vi "Write Config Unitest.vi"(8 "error in (no error)":errorcluster, 11 "main ref":T1) -> (0 "error out":errorcluster)   [LabVIEW 2025]
uses:
  controls/LAB-IQ UI Data.ctl
  Config file  FGV Unitest enum.ctl
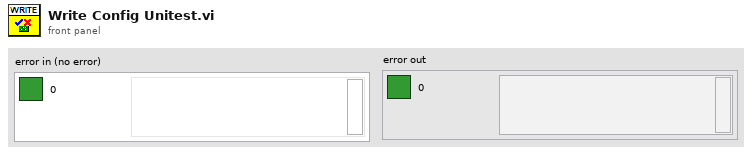
[diagram p1: front panel]
types:
  T1 = typedef "LAB-IQ UI Data.ctl" = cluster{"Main Home Screen":cluster{"GUI":refnum<vi>, "Platform Settings":refnum<vi>, "Configure":refnum<vi>, "Home":refnum<vi>, "EXIT":refnum<vi>, "service 2":refnum<vi>, "MainPage":refnum<vi>, "Analysis":refnum<vi>}, "Platform Settings":cluster{"mm/s  Surge":refnum<vi>, "Update Surge Speed":refnum<vi>, "Drive Error":refnum<vi>, "Disable Axis Jog Soft Limits":refnum<vi>, "mm/s  Sway":refnum<vi>, "Sway and Surge COM Status":refnum<vi>, "Heave COM Status":refnum<vi>, "Enable Platform":refnum<vi>, "Surge Forward Main":refnum<vi>, "Sway Right Main":refnum<vi>, "Sway Left Main":refnum<vi>, "Heave Down Main":refnum<vi>, "Heave Up main":refnum<vi>, "Update Sway Speed":refnum<vi>, "Update Heave Speed":refnum<vi>, "mm/s Heave":refnum<vi>, "mm/sec":refnum<vi>, "mm":refnum<vi>, "Surge Backward Main":refnum<vi>}, "Analysis Screen":cluster{"Analysis Home":refnum<vi>, "Surface Analysis":refnum<vi>, "Imaging":refnum<vi>, "Image Analysis":refnum<vi>, "Post Analysis":refnum<vi>}, "Config Screen":cluster{"Select Load Head":refnum<vi>, "Notes :":refnum<vi>, "FILE":refnum<vi>, "Sample ID :":refnum<vi>, "Operator ID :":refnum<vi>, "Operator Name :":refnum<vi>, "Auto":refnum<vi>}, "Motion Module":cluster{"zNL":refnum<vi>, "NL disp":refnum<vi>, "Rotary Tab":refnum<vi>, "Motion Direction:  3":refnum<vi>, "E.Velocity 2":refnum<vi>, "e.v/ssr 2":refnum<vi>, "Enter Fixed E.Velocity 2":refnum<vi>, "Enter Final SRR 2":refnum<vi>, "Enter initial SRR 2":refnum<vi>, "Enter Fixed SRR 2":refnum<vi>, "Enter the Final E.Velocity (m/s) 2":refnum<vi>, "Enter initial E.Velocity (m/s) 2":refnum<vi>, "Final Speed (RPM) 3":refnum<vi>, "Initial Speed (RPM) 2":refnum<vi>, "Enter the Final Velocity (m/s) 3":refnum<vi>, "Enter initial Velocity (m/s)  3":refnum<vi>, "Ramp Up 2":refnum<vi>, "TEST SELECTION":refnum<vi>, "SPEED SELECTION : ":refnum<vi>, "Angular Oscillation Set":refnum<vi>, "Traction":refnum<vi>, "Step Speed":refnum<vi>, "StepTable For Load-Speed":refnum<vi>, "StepTable For Speed":refnum<vi>, "Surge Forward MM":refnum<vi>, "Surge Backward MM":refnum<vi>, "M3 Image":refnum<vi>, "String 39":refnum<vi>, "Sway Left MM":refnum<vi>, "Sway Right MM":refnum<vi>, "Disable Axis Jog Soft Limits":refnum<vi>, "mm":refnum<vi>, "Heave Down MM":refnum<vi>, "Heave Up MM":refnum<vi>, "Wear Track Diameter (mm)":refnum<vi>, "Set WTD":refnum<vi>, "HomeScratch":refnum<vi>, "HomeRot":refnum<vi>, "PlaceModule":refnum<vi>, "Enter the Angle (Deg)":refnum<vi>, "Enter the Frequency (Hz)":refnum<vi>, "Motion Mode:":refnum<vi>, "LR Sway":refnum<vi>, "Rot Hor":refnum<vi>, "Scratch":refnum<vi>, "LR Cam":refnum<vi>, "MMBack":refnum<vi>, "MMNext":refnum<vi>, "Rot Ver":refnum<vi>, "Rotary Module Selection":refnum<vi>, "calculate rotary":refnum<vi>, "SPEED SELECTION : rotary":refnum<vi>, "Import 2":refnum<vi>, "Save 2":refnum<vi>, "File Path :  2":refnum<vi>, "String 45":refnum<vi>, "StepTable For Speed 3":refnum<vi>, "Enter the Speed(mm/sec)":refnum<vi>, "Enter the Speed(RPM)":refnum<vi>, "Enter Scratch Speed (mm/s):":refnum<vi>, "SwaySpeed Set":refnum<vi>, "Scartch Offset":refnum<vi>, "Motion type:":refnum<vi>, "HomeScratch 2":refnum<vi>, "Enter Scratch length (mm):":refnum<vi>, "Wear Track Diameter":refnum<vi>, "Rotary Speed Exced":refnum<vi>, "Scratch Mode":refnum<vi>, "No of Scratch":refnum<vi>}, "Environmental control":cluster{"Humidity  Status  3":refnum<vi>, "Low Temp  Status  2":refnum<vi>, "TK4 status 2":refnum<vi>, "Stage Temperature":refnum<vi>, "Sample Temperature":refnum<vi>, "Humidity (Amb)":refnum<vi>, "Clear List":refnum<vi>, "Add to list":refnum<vi>, "Wear":refnum<vi>, "Vibration":refnum<vi>, "Humidity (Chamber)":refnum<vi>, "Temperature (Chamber)":refnum<vi>, "ECR ":refnum<vi>, "Temperature (Amb)":refnum<vi>, "Microphone":refnum<vi>, "Acoustic Emission 3":refnum<vi>, "SNext":refnum<vi>, "APBack":refnum<vi>, "Enter the Temperature (°C):":refnum<vi>, "Enter the Stage \nTemperature (°C):":refnum<vi>, "Enter the Humidity (%Rh):":refnum<vi>, "Low Temp":refnum<vi>, "High Temp":refnum<vi>, "Humidity":refnum<vi>, "Sensors Picked":refnum<vi>}, "About Screen":cluster{"Password":refnum<vi>, "Home Service":refnum<vi>, "Advanced Setting":refnum<vi>, "About Tab":refnum<vi>, "ECR Port:":refnum<vi>, "Ramp Port:":refnum<vi>, "Installation/Replacement completed":refnum<vi>, "Loahead":refnum<vi>, "Heave and Surge COM Port:":refnum<vi>, "Sway COM Port:":refnum<vi>, "Temp Modbus:":refnum<vi>, "Humidity Port:":refnum<vi>, "Edit Gain Constants":refnum<vi>, "Save Gain Constants":refnum<vi>}, "Main Screen":cluster{"Main Screen Tab":refnum<vi>, "Angle and Frequency":refnum<vi>, "Stroke (mm)":refnum<vi>, "Angle (Deg)":refnum<vi>, "Main Speed Tab":refnum<vi>, "MTM MOTOR DISPLAY":refnum<vi>, "Disc Speed (m/sec)":refnum<vi>, "Ball Speed (m/sec)":refnum<vi>, "Disc Speed (RPM)":refnum<vi>, "Ball Speed (RPM)":refnum<vi>, "SPEED TAB":refnum<vi>, "Speed (m/sec)":refnum<vi>, "Set Speed (m/sec)":refnum<vi>, "Speed (RPM)":refnum<vi>, "Set Speed":refnum<vi>, "Time Tab":refnum<vi>, "Time ( HH:MM:SS ) 2":refnum<vi>, "Test Duration":refnum<vi>, "Test Duration 4":refnum<vi>, "TEST CYCLE":refnum<vi>, "TOTAL CYCLES":refnum<vi>, "Set Load (N)":refnum<vi>, "Temp Tabs":refnum<vi>, "Heater":refnum<vi>, "TK4 status":refnum<vi>, "ChamberTemp":refnum<vi>, "SetTmp":refnum<vi>, "Controller  Status":refnum<vi>, "ChamberTemp 2":refnum<vi>, "SetTmp 2":refnum<vi>, "Controller  Status 2":refnum<vi>, "ChamberTemp 3":refnum<vi>, "SetTmp 3":refnum<vi>, "Cooling":refnum<vi>, "Load Communication":refnum<vi>, "Ambient \nTemperature":refnum<vi>, "HumCOMStatus":refnum<vi>, "Ambient\n Humidity":refnum<vi>, "Freq (Hz)":refnum<vi>, "Load En":refnum<vi>, "NLt":refnum<vi>, "zNL 2":refnum<vi>, "Humidity On":refnum<vi>, "humidity disp":refnum<vi>, "Set Humidity":refnum<vi>, "NL disp 2":refnum<vi>, "Humidity On 2":refnum<vi>, "humidity disp 2":refnum<vi>, "Set Humidity 2":refnum<vi>, "NL disp 3":refnum<vi>, "AppLoadSeq scratch":refnum<vi>, "Stop Scratch":refnum<vi>, "ClrLog":refnum<vi>, "Trip Log":refnum<vi>, "STOP":refnum<vi>, "Start Test":refnum<vi>, "Test status":refnum<vi>, "AR Led":refnum<vi>, "Data":refnum<vi>, "Health":refnum<vi>, "Sway COM Status":refnum<vi>, "Heave COM Status":refnum<vi>, "Grp Tab":refnum<vi>, "Sub Graph":refnum<vi>, "SD (mm)":refnum<vi>, "Siliding distance Reset Graph":refnum<vi>, "SDGp":refnum<vi>, "Humidity Reset Graph":refnum<vi>, "HumrGp":refnum<vi>, "Acoustic Emission (mV)":refnum<vi>, "Aqucostic Reset Graph":refnum<vi>, "gACQUOS":refnum<vi>, "ECR RESET":refnum<vi>, "ECR":refnum<vi>, "Temperature Reset":refnum<vi>, "Acoustic Emission (mV) 2":refnum<vi>, "Aqucostic Reset Graph 2":refnum<vi>, "gACQUOS 2":refnum<vi>, "ECR RESET 2":refnum<vi>, "ECR 2":refnum<vi>, "Temperature Reset 2":refnum<vi>, "Temperature (deg c)":refnum<vi>, "Speed Reset Graph":refnum<vi>, "Speed Tab":refnum<vi>, "MTM DISC  SPEED":refnum<vi>, "MTM BALL SPEED":refnum<vi>, "speed mm/sec":refnum<vi>, "Hymidity":refnum<vi>, "Humidity Disable trip":refnum<vi>, "CoF Trip  2":refnum<vi>, "Depth Trip":refnum<vi>, "Weart Deapth":refnum<vi>, "Depth Reset Graph":refnum<vi>, "Weart":refnum<vi>, "Depthz":refnum<vi>, "Depth (µm)":refnum<vi>, "WearGp":refnum<vi>, "NL Trip 2":refnum<vi>, "Load pid":refnum<vi>, "Load Disable Trip":refnum<vi>, "Load Reset Graph":refnum<vi>, "NL Display 4":refnum<vi>, "Main Chart 3":refnum<vi>, "BACK":refnum<vi>, "Depth Trip 2":refnum<vi>, "COF TRIP ":refnum<vi>, "Friction Force (N)":refnum<vi>, "FF Reset Graph":refnum<vi>, "FF Disable Trip":refnum<vi>, "FF TRIP":refnum<vi>, "COF Disable Trip":refnum<vi>, "COF Reset Graph":refnum<vi>, "Start Test Temp":refnum<vi>, "zFF":refnum<vi>, "Friction Force (N) Graph":refnum<vi>, "Coefficient of Friction":refnum<vi>, "Scratch Start Test":refnum<vi>, "FF Tab":refnum<vi>, "Cyclic Friction Force (N)":refnum<vi>, "CZ FF":refnum<vi>, "Cyclic Friction Force (N) Graph":refnum<vi>, "Cyclic Coefficient of Friction":refnum<vi>, "Cyclic FF TRIP":refnum<vi>, "Cyclic FF Disable Trip":refnum<vi>, "cyclic COF Disable Trip":refnum<vi>, "cyclic COF TRIP":refnum<vi>, "cyclic COF Reset Graph":refnum<vi>, "Cyclic FF Reset Graph":refnum<vi>, "Test Trip":refnum<vi>, "Multi Scratch Pass":refnum<vi>, "Scratch Start Recording":refnum<vi>}, "Loading":cluster{"Indentation":refnum<vi>, "Reference Sample":refnum<vi>, "Load Cell Communication Slide":refnum<vi>, "com 3":refnum<vi>, "com":refnum<vi>, "DecaForce COM Status":refnum<vi>, "Update":refnum<vi>, "Clear 3":refnum<vi>, "seq":refnum<vi>, "Stribeck table":refnum<vi>, "Stribeck Table  For loading":refnum<vi>, "Loading Mode":refnum<vi>, "Enter the Final Load (N)":refnum<vi>, "Enter the CoF Trip":refnum<vi>, "Enter the Friction Force Trip":refnum<vi>, "Enter the Normal load Trip":refnum<vi>, "Enter the Load  (N)":refnum<vi>, "KiloForce":refnum<vi>, "DecaForce ":refnum<vi>, "MicroForce":refnum<vi>, "LHBack":refnum<vi>, "LHNext":refnum<vi>, "Enter the Loading Rate (N/min)":refnum<vi>, "Message":refnum<vi>, "Warning 2":refnum<vi>, "SSP 0.75":refnum<vi>, "SSP 0.5":refnum<vi>, "SSP 0.3":refnum<vi>, "Warning":refnum<vi>, "gui GIF":refnum<vi>, "Communication is established":refnum<vi>, "AppLoad 4":refnum<vi>, "Multipoint":refnum<vi>, "Load Selection":refnum<vi>}, "PID":cluster{"Ramp MulFac":refnum<vi>, "pulses LoadDiffRamp(2..10)":refnum<vi>, "PulseControlRamp(diff<=3N)":refnum<vi>, "SetLoadDeadband(%) Load(0-10N)":refnum<vi>, "PID gains out delay (microForce)":refnum<vi>, "Ramp":refnum<vi>, "Gain 2":refnum<vi>, "pulses LoadDiff(2..10)":refnum<vi>, "pulses LoadDiff(11..50)":refnum<vi>, "PulseControl(diff<=3N)":refnum<vi>, "SetLoadDeadband(%)  2":refnum<vi>, "Dummy Run":refnum<vi>, "Vertical load (N)":refnum<vi>, "AutoTune":refnum<vi>, "Offset 3 ":refnum<vi>, "apply load":refnum<vi>, "Offset  3":refnum<vi>, "apply load 2":refnum<vi>, "Enter ByPass Load":refnum<vi>, "reinit 3":refnum<vi>, "output range delay":refnum<vi>, "PID gains out delay":refnum<vi>, "Bypass Load":refnum<vi>, "pulsesSent":refnum<vi>, "pulses ":refnum<vi>, "actpid":refnum<vi>, "gFF Rot":refnum<vi>, "pulses LoadDiff(21..1000)":refnum<vi>, "Delay":refnum<vi>, "deadband":refnum<vi>}, "Config Parameters":cluster{"Tab Control 3":refnum<vi>, "Tab Control 19":refnum<vi>, "SAMPLES":refnum<vi>, "Re-initilaize":refnum<vi>, "Filter ON/OFF":refnum<vi>, "TracHomeSurgeOffsetCounts 10MM":refnum<vi>, "TracHomeSwayOffsetCounts 10MM":refnum<vi>, "Acoustic Emission:":refnum<vi>, "Apply Filter (FF)":refnum<vi>, "Filter% 2":refnum<vi>, "Apply Filter (Load)":refnum<vi>, "Filter% ":refnum<vi>, "Sway distance (mm)":refnum<vi>, "Surge distance (mm)":refnum<vi>, "DataSavingLoopDelay(ms)":refnum<vi>, "SAVE 2":refnum<vi>, "Enter Distance":refnum<vi>, "Sway Counts:":refnum<vi>, "Distance (mm): 3":refnum<vi>, "Surge Counts:":refnum<vi>, "Distance (mm): 2":refnum<vi>, "Distance (mm):":refnum<vi>, "Heave Counts:":refnum<vi>, "LRMHomeSurgeOffsetCounts":refnum<vi>, "LRMHomeSwayOffsetCounts":refnum<vi>, "TracHomeSurgeOffsetCounts 20MM":refnum<vi>, "TracHomeSwayOffsetCounts 20MM":refnum<vi>, "RotHomeSwayOffsetCounts":refnum<vi>, "RotHomeSurgeOffsetCounts":refnum<vi>, "Heave distance":refnum<vi>, "Zmm":refnum<vi>, "Heave Pulses/mm":refnum<vi>, "Surge Pulses/mm":refnum<vi>, "Sway Pulses/mm":refnum<vi>, "Heave Pitch":refnum<vi>, "Surge Pitch":refnum<vi>, "Sway Pitch":refnum<vi>, "Heave PPR":refnum<vi>, "Surge PPR":refnum<vi>, "Sway PPR":refnum<vi>, "Tab Control 5":refnum<vi>, "Tab Control 14":refnum<vi>, "Tab Control 26":refnum<vi>, "AE":refnum<vi>, "Heave Loop Delay":refnum<vi>, "Heave PID Speed":refnum<vi>, "Surge Jog Speed":refnum<vi>, "Heave Jog Speed":refnum<vi>, "Sway Loop Delay":refnum<vi>, "Sway PID Speed":refnum<vi>, "Sway Jog Speed":refnum<vi>, "DEPTH TRIP VALUE":refnum<vi>, "LOAD TRIP VALUE":refnum<vi>, "DEPTH TRIP   ENABLE":refnum<vi>, "LOAD TRIP  ENABLE":refnum<vi>, "CYCLIC FF TRIP VALUE":refnum<vi>, "FF TRIP VALUE":refnum<vi>, "CYCLIC CoF TRIP VALUE":refnum<vi>, "COF TRIP VALUE":refnum<vi>, "CYCLIC COF TRIP  ENABLE":refnum<vi>, "CYCLIC FF TRIP  ENABLE":refnum<vi>, "FF TRIP  ENABLE":refnum<vi>, "COF TRIP  ENABLE":refnum<vi>}, "Loading Com Port":cluster{"ClearAll":refnum<vi>, "Mz(Nm)":refnum<vi>, "My(Nm)":refnum<vi>, "Mx(Nm)":refnum<vi>, "Save Dwell":refnum<vi>, "Mx ":refnum<vi>, "My ":refnum<vi>, "Mz":refnum<vi>, "Fx(N)":refnum<vi>, "Fy(N)":refnum<vi>, "Fz(N)":refnum<vi>, "ZeroAll":refnum<vi>, "Acq Delay (ms)":refnum<vi>, "Burst Delay (ms)":refnum<vi>, "model":refnum<vi>, "SN":refnum<vi>, "FFx(N)":refnum<vi>, "Sensor IP":refnum<vi>, "Port":refnum<vi>, "FFy(N)":refnum<vi>, "Load(N)":refnum<vi>, "delete Handle":refnum<vi>, "Create Handle":refnum<vi>, "ft_data":refnum<vi>, "ft_range":refnum<vi>, "ft_data 2":refnum<vi>, "stop 6":refnum<vi>, "running_flag":refnum<vi>, "ft_udp_handle":refnum<vi>, "get-data-return":refnum<vi>, "get-range-return":refnum<vi>, "zero-return":refnum<vi>, "filter-return":refnum<vi>, "initial-return":refnum<vi>, "deleteHandle-result":refnum<vi>, "Load Cell Temp":refnum<vi>}, "Heave AND Surge":cluster{"SURGE POSE":refnum<vi>, "error out Read":refnum<vi>, "HEAVE POSE":refnum<vi>, "State":refnum<vi>, "Homed":refnum<vi>, "Sequence ID":refnum<vi>, "error out Write":refnum<vi>, "faultCode":refnum<vi>, "Ack ID":refnum<vi>, "SPEED":refnum<vi>, "Distance":refnum<vi>, "Mode Command":refnum<vi>, "Heave and Surge Read":refnum<vi>, "Read Heave Temp":refnum<vi>, "Spare 15":refnum<vi>, "Spare 14":refnum<vi>, "Spare 13":refnum<vi>, "Spare 12":refnum<vi>, "Spare 11":refnum<vi>, "Spare 10":refnum<vi>, "Spare 9":refnum<vi>, "Spare 8":refnum<vi>, "Spare 7":refnum<vi>, "Spare 6":refnum<vi>, "Spare 5":refnum<vi>, "Spare 4":refnum<vi>, "Spare 2":refnum<vi>, "Spare 1":refnum<vi>, "Node Id":refnum<vi>, "Spare 3":refnum<vi>, "SPARE 4":refnum<vi>, "SPARE 3":refnum<vi>, "SPARE 2":refnum<vi>, "SPARE 1":refnum<vi>, "fwMajor":refnum<vi>, "fwMinor":refnum<vi>, "Manual Write":refnum<vi>, "Heave and Surge Write":refnum<vi>}, "New PID LOGIC":cluster{"Fine Tune Zone":refnum<vi>, "PID SDelay":refnum<vi>, "Max_pos_limit":refnum<vi>, "Min_pos_limit":refnum<vi>, "i_limit":refnum<vi>, "pct_scale":refnum<vi>, "Deadband":refnum<vi>, "Kd":refnum<vi>, "Ki":refnum<vi>, "Kp":refnum<vi>, "Current Position":refnum<vi>, "Set Load":refnum<vi>, "Current Load":refnum<vi>, "Pulse delta":refnum<vi>, "Init Step":refnum<vi>, "Max Step Linit":refnum<vi>}, "SWAY ":cluster{"fwMajor":refnum<vi>, "Homed":refnum<vi>, "Rotary POSE":refnum<vi>, "State":refnum<vi>, "SWAY POSE":refnum<vi>, "Ack ID":refnum<vi>, "faultCode":refnum<vi>, "Node Id":refnum<vi>, "fwMinor":refnum<vi>, "Spare 6":refnum<vi>, "Spare 5":refnum<vi>, "Spare 4":refnum<vi>, "Spare 3":refnum<vi>, "Spare 2":refnum<vi>, "Spare 1":refnum<vi>, "Spare 7":refnum<vi>, "SPARE  5":refnum<vi>, "error out Write  SWAY ":refnum<vi>, "error out Read SWAY ":refnum<vi>, "Manual Write SWAY ":refnum<vi>, "SWAY WRITE":refnum<vi>, "SPARE  4":refnum<vi>, "SPARE  3":refnum<vi>, "SPARE 2":refnum<vi>, "SPARE 1":refnum<vi>, "Spare 15":refnum<vi>, "Spare 14":refnum<vi>, "Spare 13":refnum<vi>, "Spare 12":refnum<vi>, "Spare 11":refnum<vi>, "Spare 9":refnum<vi>, "Spare 8":refnum<vi>, "SPEED":refnum<vi>, "Distance":refnum<vi>, "Mode Command":refnum<vi>, "Sequence ID":refnum<vi>, "SWAY READ":refnum<vi>, "Spare 10":refnum<vi>, "Read SWAY Temp":refnum<vi>}, "Analysis Screen":cluster{"Analysis Home":refnum<vi>, "Refresh 2":refnum<vi>, "MEAN 4":refnum<vi>, "SD 4":refnum<vi>, "VARIANCE 4":refnum<vi>, "MEAN  3":refnum<vi>, "SD  3":refnum<vi>, "VARIANCE  3":refnum<vi>, "MEAN 2":refnum<vi>, "SD  2":refnum<vi>, "VARIANCE 2":refnum<vi>, "MEAN":refnum<vi>, "SD":refnum<vi>, "VARIANCE":refnum<vi>, "File 4 Discription":refnum<vi>, "OPEN 4":refnum<vi>, "File Name 4":refnum<vi>, "OPEN 3":refnum<vi>, "File 3 Discription":refnum<vi>, "File Name 3":refnum<vi>, "Y-AXIS":refnum<vi>, "X-AXIS":refnum<vi>, "XY Graph":refnum<vi>, "File Name 2":refnum<vi>, "File Name 1":refnum<vi>, "OPEN 2":refnum<vi>, "OPEN 1":refnum<vi>, "File 1 Discription ":refnum<vi>, "File 2 Discription":refnum<vi>, "Export":refnum<vi>, "File Format":refnum<vi>}}
  T2 = typedef "Config file  FGV Unitest enum.ctl" = enum16{"OPEN", "READ", "WRITE", "CLOSE"}
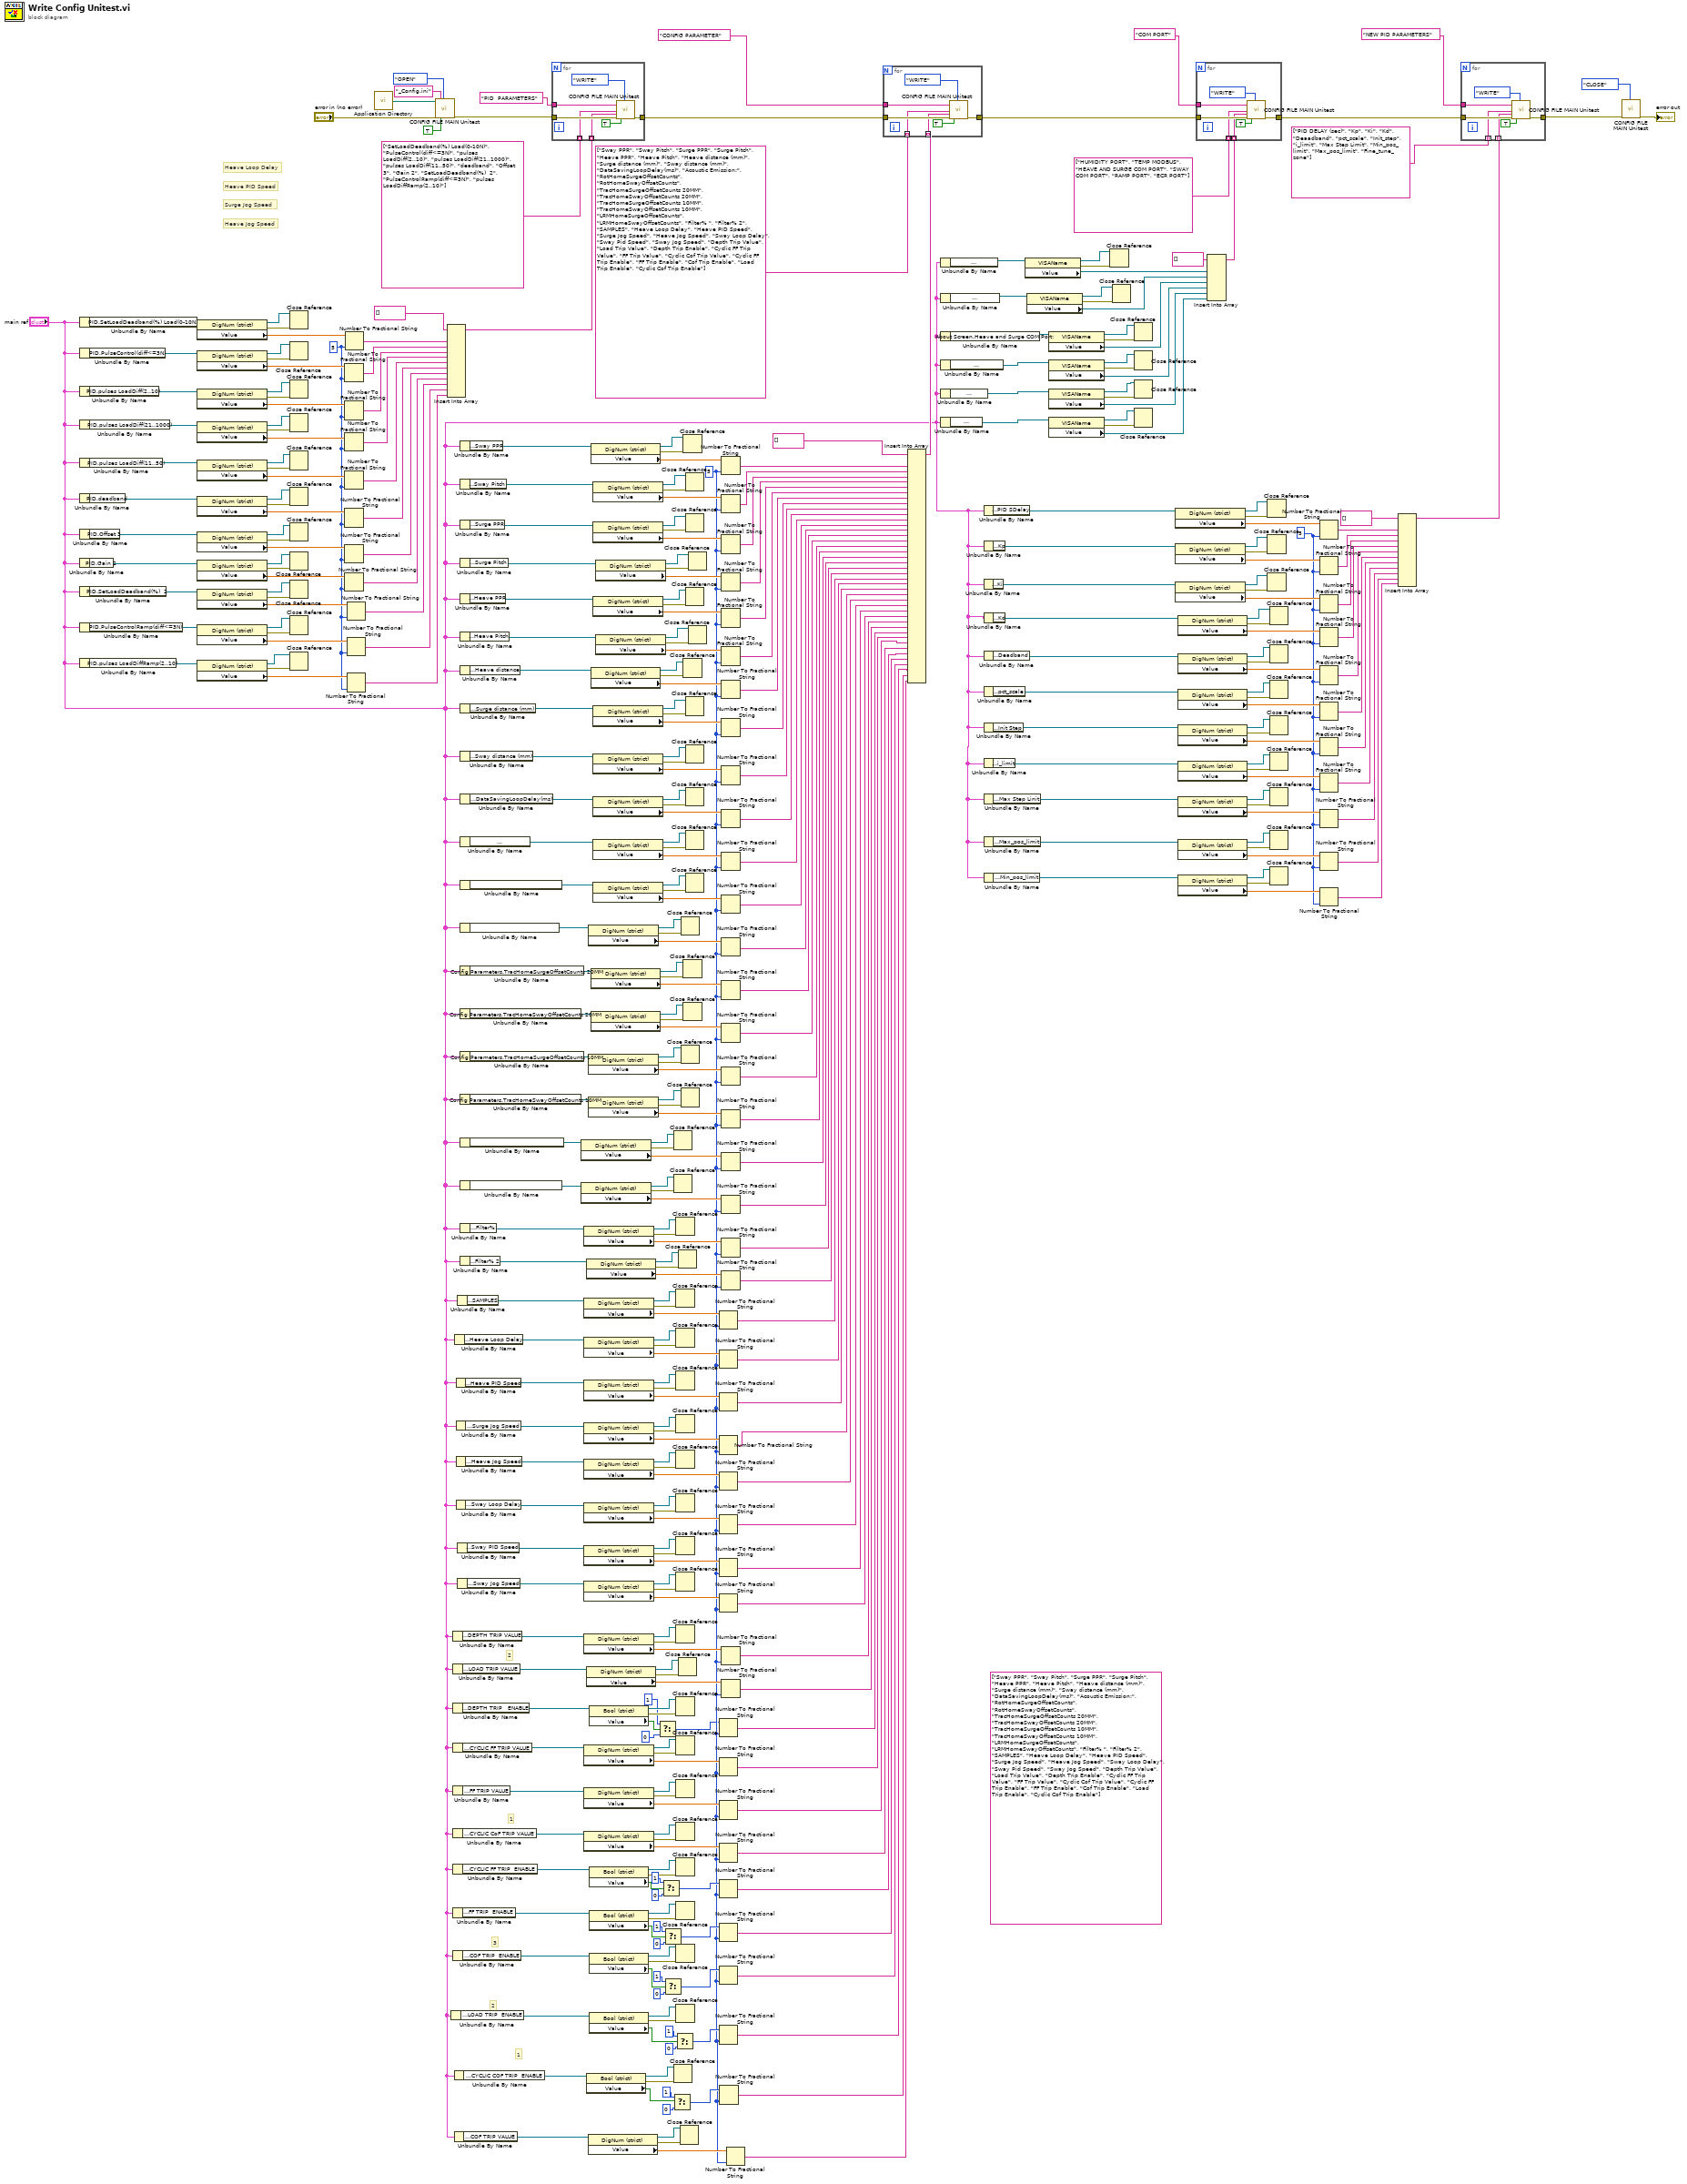
[diagram p0: block diagram]
diagram:
  (unwired) string[] ["Sway PPR", "Sway Pitch", "Surge PPR", "Surge Pitch", "Heave PPR", "Heave Pitch", "Heave distance (mm)", "Surge distance (mm)", "Sway distance (mm)", "DataSavingLoopDelay(ms)", "Acoustic Emission:", "RotHomeSurgeOffsetCounts", "RotHomeSwayOffsetCounts", "TracHomeSurgeOffsetCounts 20MM", "TracHomeSwayOffsetCounts 20MM", "TracHomeSurgeOffsetCounts 10MM", "TracHomeSwayOffsetCounts 10MM", "LRMHomeSurgeOffsetCounts", "LRMHomeSwayOffsetCounts", "Filter% ", "Filter% 2", "SAMPLES", "Heave Loop Delay", "Heave PID Speed", "Surge Jog Speed", "Heave Jog Speed", "Sway Loop Delay", "Sway Pid Speed", "Sway Jog Speed", "Depth Trip Value", "Load Trip Value", "Depth Trip Enable", "Cyclic FF Trip Value", "FF Trip Value", "Cyclic Cof Trip Value", "Cyclic FF Trip Enable", "FF Trip Enable", "Cof Trip Enable", "Load Trip Enable", "Cyclic Cof Trip Enable"]
  w110 = i16 5 ("precision (6)")
  w4 = i16 5 ("precision (6)")
  w329 = i16 5 ("precision (6)")
  # "3"
  # "2"
  # "2"
  # "1"
  # "1"
  # "Heave Jog Speed"
  # "Surge Jog Speed"
  # "Heave PID Speed"
  # "Heave Loop Delay"
  n1 = Unbundle By Name("main ref") -> ("PID.SetLoadDeadband(%) Load(0-10N)"=w373:refnum<vi>)
  n2 = Unbundle By Name("main ref") -> ("PID.PulseControl(diff<=3N)"=w368:refnum<vi>)
  n3 = Unbundle By Name("main ref") -> ("PID.pulses LoadDiff(2..10)"=w367:refnum<vi>)
  n4 = Unbundle By Name("main ref") -> ("PID.pulses LoadDiff(21..1000)"=w362:refnum<vi>)
  n5 = Unbundle By Name("main ref") -> ("PID.pulses LoadDiff(11..50)"=w361:refnum<vi>)
  n6 = Unbundle By Name("main ref") -> ("PID.deadband"=w356:refnum<vi>)
  n7 = Unbundle By Name("main ref") -> ("PID.Offset 3"=w355:refnum<vi>)
  n8 = Unbundle By Name("main ref") -> ("PID.Gain 2"=w350:refnum<vi>)
  n9 = Unbundle By Name("main ref") -> ("PID.SetLoadDeadband(%)  2"=w349:refnum<vi>)
  n10 = Unbundle By Name("main ref") -> ("PID.PulseControlRamp(diff<=3N)"=w345:refnum<vi>)
  n11 = Unbundle By Name("main ref") -> ("PID.pulses LoadDiffRamp(2..10)"=w343:refnum<vi>)
  n12 = property class="DigNum (strict)"(reference=w373) -> (reference out=w371:refnum<vi>, error out=w372:errorcluster, "Value"=w339:dbl)  [unwired: 1 in]
  n13 = property class="DigNum (strict)"(reference=w368) -> (reference out=w370:refnum<vi>, error out=w369:errorcluster, "Value"=w340:dbl)  [unwired: 1 in]
  n14 = property class="DigNum (strict)"(reference=w367) -> (reference out=w365:refnum<vi>, error out=w366:errorcluster, "Value"=w338:dbl)  [unwired: 1 in]
  n15 = property class="DigNum (strict)"(reference=w362) -> (reference out=w364:refnum<vi>, error out=w363:errorcluster, "Value"=w337:dbl)  [unwired: 1 in]
  n16 = property class="DigNum (strict)"(reference=w361) -> (reference out=w359:refnum<vi>, error out=w360:errorcluster, "Value"=w336:dbl)  [unwired: 1 in]
  n17 = property class="DigNum (strict)"(reference=w356) -> (reference out=w358:refnum<vi>, error out=w357:errorcluster, "Value"=w335:dbl)  [unwired: 1 in]
  n18 = property class="DigNum (strict)"(reference=w355) -> (reference out=w353:refnum<vi>, error out=w354:errorcluster, "Value"=w334:dbl)  [unwired: 1 in]
  n19 = property class="DigNum (strict)"(reference=w350) -> (reference out=w352:refnum<vi>, error out=w351:errorcluster, "Value"=w333:dbl)  [unwired: 1 in]
  n20 = property class="DigNum (strict)"(reference=w349) -> (reference out=w347:refnum<vi>, error out=w348:errorcluster, "Value"=w332:dbl)  [unwired: 1 in]
  n21 = property class="DigNum (strict)"(reference=w345) -> (reference out=w344:refnum<vi>, error out=w346:errorcluster, "Value"=w331:dbl)  [unwired: 1 in]
  n22 = property class="DigNum (strict)"(reference=w343) -> (reference out=w341:refnum<vi>, error out=w342:errorcluster, "Value"=w330:dbl)  [unwired: 1 in]
  n23 = Close Reference(reference=w371, error in (no error)=w372) -> ()  [unwired: 1 out]
  n24 = Close Reference(reference=w370, error in (no error)=w369) -> ()  [unwired: 1 out]
  n25 = Close Reference(reference=w365, error in (no error)=w366) -> ()  [unwired: 1 out]
  n26 = Close Reference(reference=w364, error in (no error)=w363) -> ()  [unwired: 1 out]
  n27 = Close Reference(reference=w359, error in (no error)=w360) -> ()  [unwired: 1 out]
  n28 = Close Reference(reference=w358, error in (no error)=w357) -> ()  [unwired: 1 out]
  n29 = Close Reference(reference=w353, error in (no error)=w354) -> ()  [unwired: 1 out]
  n30 = Close Reference(reference=w352, error in (no error)=w351) -> ()  [unwired: 1 out]
  n31 = Close Reference(reference=w347, error in (no error)=w348) -> ()  [unwired: 1 out]
  n32 = Close Reference(reference=w344, error in (no error)=w346) -> ()  [unwired: 1 out]
  n33 = Close Reference(reference=w341, error in (no error)=w342) -> ()  [unwired: 1 out]
  n34 = Number To Fractional String(number=w340, precision (6)=w329) -> (F-format string=w326:string)  [unwired: 2 in]
  n35 = Number To Fractional String(number=w338, precision (6)=w329) -> (F-format string=w325:string)  [unwired: 2 in]
  n36 = Number To Fractional String(number=w337, precision (6)=w329) -> (F-format string=w324:string)  [unwired: 2 in]
  n37 = Number To Fractional String(number=w336, precision (6)=w329) -> (F-format string=w323:string)  [unwired: 2 in]
  n38 = Number To Fractional String(number=w335, precision (6)=w329) -> (F-format string=w322:string)  [unwired: 2 in]
  n39 = Number To Fractional String(number=w334, precision (6)=w329) -> (F-format string=w321:string)  [unwired: 2 in]
  n40 = Number To Fractional String(number=w333, precision (6)=w329) -> (F-format string=w320:string)  [unwired: 2 in]
  n41 = Number To Fractional String(number=w339, precision (6)=w329) -> (F-format string=w327:string)  [unwired: 2 in]
  n42 = Number To Fractional String(number=w332, precision (6)=w329) -> (F-format string=w319:string)  [unwired: 2 in]
  n43 = Number To Fractional String(number=w331, precision (6)=w329) -> (F-format string=w318:string)  [unwired: 2 in]
  n44 = Number To Fractional String(number=w330, precision (6)=w329) -> (F-format string=w317:string)  [unwired: 2 in]
  n45 = call <vilib>:"Application Directory.vi"() -> ("Application Directory"=w385:path)
  n46 = call "CONFIG FILE MAIN Unitest.vi"("File Path"=w385, "error in"="error in (no error)", "file name"="_Config.ini", "PARAMETER/CONFIG"=TRUE, "Config Enum"=Config_file__FGV_Unitest_enum."OPEN") -> ("error out"=w384:errorcluster)  [unwired: 13 in, 1 out]
  n47 = Insert Into Array(array=string[] [], new element #1=w327, new element #2=w326, new element #3=w325, new element #4=w324, new element #5=w323, new element #6=w322, new element #7=w321, new element #8=w320, new element #9=w319, new element #10=w318, new element #11=w317) -> (w316:string[])  [unwired: 1 in]
  n48 = Unbundle By Name("main ref") -> ("Config Parameters.LOAD TRIP  ENABLE"=w46:refnum<vi>)
  n49 = Unbundle By Name("main ref") -> ("Config Parameters.DEPTH TRIP VALUE"=w50:refnum<vi>)
  n50 = Unbundle By Name("main ref") -> ("Config Parameters.LOAD TRIP VALUE"=w56:refnum<vi>)
  n51 = Unbundle By Name("main ref") -> ("Config Parameters.DEPTH TRIP   ENABLE"=w57:refnum<vi>)
  n52 = Unbundle By Name("main ref") -> ("Config Parameters.CYCLIC FF TRIP VALUE"=w64:refnum<vi>)
  n53 = Unbundle By Name("main ref") -> ("Config Parameters.FF TRIP VALUE"=w65:refnum<vi>)
  n54 = Unbundle By Name("main ref") -> ("Config Parameters.CYCLIC CoF TRIP VALUE"=w72:refnum<vi>)
  n55 = Unbundle By Name("main ref") -> ("Config Parameters.CYCLIC FF TRIP  ENABLE"=w73:refnum<vi>)
  n56 = Unbundle By Name("main ref") -> ("Config Parameters.FF TRIP  ENABLE"=w81:refnum<vi>)
  n57 = Unbundle By Name("main ref") -> ("Config Parameters.COF TRIP  ENABLE"=w76:refnum<vi>)
  n58 = Unbundle By Name("main ref") -> ("Config Parameters.CYCLIC COF TRIP  ENABLE"=w31:refnum<vi>)
  n59 = Unbundle By Name("main ref") -> ("Config Parameters.COF TRIP VALUE"=w9:refnum<vi>)
  n60 = Unbundle By Name("main ref") -> ("Config Parameters.Heave Loop Delay"=w175:refnum<vi>)
  n61 = Unbundle By Name("main ref") -> ("Config Parameters.Heave PID Speed"=w174:refnum<vi>)
  n62 = Unbundle By Name("main ref") -> ("Config Parameters.Surge Jog Speed"=w167:refnum<vi>)
  n63 = Unbundle By Name("main ref") -> ("Config Parameters.Heave Jog Speed"=w166:refnum<vi>)
  n64 = Unbundle By Name("main ref") -> ("Config Parameters.Sway Loop Delay"=w85:refnum<vi>)
  n65 = Unbundle By Name("main ref") -> ("Config Parameters.SAMPLES"=w233:refnum<vi>)
  n66 = Unbundle By Name("main ref") -> ("Config Parameters.Sway PID Speed"=w92:refnum<vi>)
  n67 = Unbundle By Name("main ref") -> ("Config Parameters.Sway Jog Speed"=w93:refnum<vi>)
  n68 = Unbundle By Name("main ref") -> ("Config Parameters.Sway PPR"=w315:refnum<vi>)
  n69 = Unbundle By Name("main ref") -> ("Config Parameters.Sway Pitch"=w308:refnum<vi>)
  n70 = Unbundle By Name("main ref") -> ("Config Parameters.Surge PPR"=w300:refnum<vi>)
  n71 = Unbundle By Name("main ref") -> ("Config Parameters.Surge Pitch"=w307:refnum<vi>)
  n72 = Unbundle By Name("main ref") -> ("Config Parameters.Heave PPR"=w299:refnum<vi>)
  n73 = Unbundle By Name("main ref") -> ("Config Parameters.Heave Pitch"=w293:refnum<vi>)
  n74 = Unbundle By Name("main ref") -> ("Config Parameters.Heave distance"=w285:refnum<vi>)
  n75 = Unbundle By Name("main ref") -> ("Config Parameters.Surge distance (mm)"=w291:refnum<vi>)
  n76 = Unbundle By Name("main ref") -> ("Config Parameters.Sway distance (mm)"=w282:refnum<vi>)
  n77 = Unbundle By Name("main ref") -> ("Config Parameters.DataSavingLoopDelay(ms)"=w279:refnum<vi>)
  n78 = Unbundle By Name("main ref") -> ("Config Parameters.Acoustic Emission:"=w274:refnum<vi>)
  n79 = Unbundle By Name("main ref") -> ("Config Parameters.RotHomeSurgeOffsetCounts"=w271:refnum<vi>)
  n80 = Unbundle By Name("main ref") -> ("Config Parameters.RotHomeSwayOffsetCounts"=w266:refnum<vi>)
  n81 = Unbundle By Name("main ref") -> ("Config Parameters.TracHomeSurgeOffsetCounts 20MM"=w263:refnum<vi>)
  n82 = Unbundle By Name("main ref") -> ("Config Parameters.TracHomeSwayOffsetCounts 20MM"=w258:refnum<vi>)
  n83 = Unbundle By Name("main ref") -> ("Config Parameters.TracHomeSurgeOffsetCounts 10MM"=w252:refnum<vi>)
  n84 = Unbundle By Name("main ref") -> ("Config Parameters.TracHomeSwayOffsetCounts 10MM"=w257:refnum<vi>)
  n85 = Unbundle By Name("main ref") -> ("Config Parameters.LRMHomeSurgeOffsetCounts"=w246:refnum<vi>)
  n86 = Unbundle By Name("main ref") -> ("Config Parameters.LRMHomeSwayOffsetCounts"=w241:refnum<vi>)
  n87 = Unbundle By Name("main ref") -> ("Config Parameters.Filter%"=w240:refnum<vi>)
  n88 = Unbundle By Name("main ref") -> ("Config Parameters.Filter% 2"=w234:refnum<vi>)
  n89 = for {
    tunnel: w384 -> [w396]
    tunnel: "PID  PARAMETERS" ("WRITE /READ SECTION") -> [w395]
    tunnel: string[] ["SetLoadDeadband(%) Load(0-10N)", "PulseControl(diff<=3N)", "pulses LoadDiff(2..10)", "pulses LoadDiff(21..1000)", "pulses LoadDiff(11..50)", "deadband", "Offset  3", "Gain 2", "SetLoadDeadband(%)  2", "PulseControlRamp(diff<=3N)", "pulses LoadDiffRamp(2..10)"] -> [w392] mode=indexing
    tunnel: [w394] -> w381
    tunnel: w316 -> [w391] mode=indexing
    n90 = call "CONFIG FILE MAIN Unitest.vi"("WRITE /READ SECTION"=w395, "WRITE KEY"=w392, "WRITE VALUE"=w391, "error in"=w396, "PARAMETER/CONFIG"=TRUE, "Config Enum"=Config_file__FGV_Unitest_enum."WRITE") -> ("error out"=w394:errorcluster)  [unwired: 12 in, 1 out]
  }
  n91 = property class="DigNum (strict)"(reference=w246) -> (reference out=w247:refnum<vi>, error out=w245:errorcluster, "Value"=w244:dbl)  [unwired: 1 in]
  n92 = property class="DigNum (strict)"(reference=w241) -> (reference out=w248:refnum<vi>, error out=w242:errorcluster, "Value"=w243:dbl)  [unwired: 1 in]
  n93 = property class="DigNum (strict)"(reference=w240) -> (reference out=w237:refnum<vi>, error out=w239:errorcluster, "Value"=w238:dbl)  [unwired: 1 in]
  n94 = property class="DigNum (strict)"(reference=w233) -> (reference out=w230:refnum<vi>, error out=w232:errorcluster, "Value"=w231:dbl)  [unwired: 1 in]
  n95 = property class="DigNum (strict)"(reference=w175) -> (reference out=w178:refnum<vi>, error out=w176:errorcluster, "Value"=w177:dbl)  [unwired: 1 in]
  n96 = property class="DigNum (strict)"(reference=w174) -> (reference out=w171:refnum<vi>, error out=w173:errorcluster, "Value"=w172:dbl)  [unwired: 1 in]
  n97 = property class="DigNum (strict)"(reference=w167) -> (reference out=w170:refnum<vi>, error out=w168:errorcluster, "Value"=w169:dbl)  [unwired: 1 in]
  n98 = property class="DigNum (strict)"(reference=w166) -> (reference out=w163:refnum<vi>, error out=w165:errorcluster, "Value"=w164:dbl)  [unwired: 1 in]
  n99 = property class="DigNum (strict)"(reference=w85) -> (reference out=w88:refnum<vi>, error out=w86:errorcluster, "Value"=w87:dbl)  [unwired: 1 in]
  n100 = property class="DigNum (strict)"(reference=w92) -> (reference out=w89:refnum<vi>, error out=w91:errorcluster, "Value"=w90:dbl)  [unwired: 1 in]
  n101 = property class="DigNum (strict)"(reference=w93) -> (reference out=w96:refnum<vi>, error out=w94:errorcluster, "Value"=w95:dbl)  [unwired: 1 in]
  n102 = property class="DigNum (strict)"(reference=w50) -> (reference out=w53:refnum<vi>, error out=w51:errorcluster, "Value"=w52:dbl)  [unwired: 1 in]
  n103 = property class="DigNum (strict)"(reference=w64) -> (reference out=w61:refnum<vi>, error out=w63:errorcluster, "Value"=w62:dbl)  [unwired: 1 in]
  n104 = property class="DigNum (strict)"(reference=w65) -> (reference out=w68:refnum<vi>, error out=w66:errorcluster, "Value"=w67:dbl)  [unwired: 1 in]
  n105 = property class="DigNum (strict)"(reference=w72) -> (reference out=w69:refnum<vi>, error out=w71:errorcluster, "Value"=w70:dbl)  [unwired: 1 in]
  n106 = property class="DigNum (strict)"(reference=w234) -> (reference out=w229:refnum<vi>, error out=w235:errorcluster, "Value"=w236:dbl)  [unwired: 1 in]
  n107 = property class="DigNum (strict)"(reference=w56) -> (reference out=w60:refnum<vi>, error out=w55:errorcluster, "Value"=w54:dbl)  [unwired: 1 in]
  n108 = property class="Bool (strict)"(reference=w31) -> (reference out=w33:refnum<vi>, error out=w32:errorcluster, "Value"=w22:bool)  [unwired: 1 in]
  n109 = property class="DigNum (strict)"(reference=w9) -> (reference out=w7:refnum<vi>, error out=w8:errorcluster, "Value"=w5:dbl)  [unwired: 1 in]
  n110 = property class="DigNum (strict)"(reference=w266) -> (reference out=w265:refnum<vi>, error out=w267:errorcluster, "Value"=w268:dbl)  [unwired: 1 in]
  n111 = property class="DigNum (strict)"(reference=w252) -> (reference out=w250:refnum<vi>, error out=w253:errorcluster, "Value"=w254:dbl)  [unwired: 1 in]
  n112 = property class="DigNum (strict)"(reference=w257) -> (reference out=w249:refnum<vi>, error out=w256:errorcluster, "Value"=w255:dbl)  [unwired: 1 in]
  n113 = property class="Bool (strict)"(reference=w57) -> (reference out=w59:refnum<vi>, error out=w58:errorcluster, "Value"=w49:bool)  [unwired: 1 in]
  n114 = property class="Bool (strict)"(reference=w73) -> (reference out=w75:refnum<vi>, error out=w74:errorcluster, "Value"=w27:bool)  [unwired: 1 in]
  n115 = property class="Bool (strict)"(reference=w81) -> (reference out=w79:refnum<vi>, error out=w80:errorcluster, "Value"=w28:bool)  [unwired: 1 in]
  n116 = property class="Bool (strict)"(reference=w76) -> (reference out=w78:refnum<vi>, error out=w77:errorcluster, "Value"=w29:bool)  [unwired: 1 in]
  n117 = property class="Bool (strict)"(reference=w46) -> (reference out=w44:refnum<vi>, error out=w45:errorcluster, "Value"=w30:bool)  [unwired: 1 in]
  n118 = property class="DigNum (strict)"(reference=w315) -> (reference out=w313:refnum<vi>, error out=w314:errorcluster, "Value"=w312:dbl)  [unwired: 1 in]
  n119 = property class="DigNum (strict)"(reference=w285) -> (reference out=w204:refnum<vi>, error out=w286:errorcluster, "Value"=w287:dbl)  [unwired: 1 in]
  n120 = property class="DigNum (strict)"(reference=w263) -> (reference out=w264:refnum<vi>, error out=w262:errorcluster, "Value"=w261:dbl)  [unwired: 1 in]
  n121 = property class="DigNum (strict)"(reference=w258) -> (reference out=w251:refnum<vi>, error out=w259:errorcluster, "Value"=w260:dbl)  [unwired: 1 in]
  n122 = property class="DigNum (strict)"(reference=w308) -> (reference out=w310:refnum<vi>, error out=w309:errorcluster, "Value"=w311:dbl)  [unwired: 1 in]
  n123 = property class="DigNum (strict)"(reference=w300) -> (reference out=w302:refnum<vi>, error out=w301:errorcluster, "Value"=w303:dbl)  [unwired: 1 in]
  n124 = property class="DigNum (strict)"(reference=w299) -> (reference out=w292:refnum<vi>, error out=w298:errorcluster, "Value"=w297:dbl)  [unwired: 1 in]
  n125 = property class="DigNum (strict)"(reference=w291) -> (reference out=w289:refnum<vi>, error out=w290:errorcluster, "Value"=w288:dbl)  [unwired: 1 in]
  n126 = property class="DigNum (strict)"(reference=w282) -> (reference out=w281:refnum<vi>, error out=w283:errorcluster, "Value"=w284:dbl)  [unwired: 1 in]
  n127 = property class="DigNum (strict)"(reference=w279) -> (reference out=w280:refnum<vi>, error out=w278:errorcluster, "Value"=w277:dbl)  [unwired: 1 in]
  n128 = property class="DigNum (strict)"(reference=w274) -> (reference out=w273:refnum<vi>, error out=w275:errorcluster, "Value"=w276:dbl)  [unwired: 1 in]
  n129 = property class="DigNum (strict)"(reference=w271) -> (reference out=w272:refnum<vi>, error out=w270:errorcluster, "Value"=w269:dbl)  [unwired: 1 in]
  n130 = property class="DigNum (strict)"(reference=w307) -> (reference out=w305:refnum<vi>, error out=w306:errorcluster, "Value"=w304:dbl)  [unwired: 1 in]
  n131 = property class="DigNum (strict)"(reference=w293) -> (reference out=w295:refnum<vi>, error out=w294:errorcluster, "Value"=w296:dbl)  [unwired: 1 in]
  n132 = Select(t=1, s=w49, f=0) -> (s? t:f=w1:i32)
  n133 = Select(t=1, s=w27, f=0) -> (s? t:f=w26:i32)
  n134 = Select(t=1, s=w28, f=0) -> (s? t:f=w25:i32)
  n135 = Select(t=1, s=w29, f=0) -> (s? t:f=w24:i32)
  n136 = Select(t=1, s=w22, f=0) -> (s? t:f=w21:i32)
  n137 = Close Reference(reference=w247, error in (no error)=w245) -> ()  [unwired: 1 out]
  n138 = Close Reference(reference=w248, error in (no error)=w242) -> ()  [unwired: 1 out]
  n139 = Close Reference(reference=w33, error in (no error)=w32) -> ()  [unwired: 1 out]
  n140 = Select(t=1, s=w30, f=0) -> (s? t:f=w23:i32)
  n141 = Close Reference(reference=w237, error in (no error)=w239) -> ()  [unwired: 1 out]
  n142 = Close Reference(reference=w230, error in (no error)=w232) -> ()  [unwired: 1 out]
  n143 = Close Reference(reference=w178, error in (no error)=w176) -> ()  [unwired: 1 out]
  n144 = Close Reference(reference=w171, error in (no error)=w173) -> ()  [unwired: 1 out]
  n145 = Close Reference(reference=w170, error in (no error)=w168) -> ()  [unwired: 1 out]
  n146 = Close Reference(reference=w163, error in (no error)=w165) -> ()  [unwired: 1 out]
  n147 = Close Reference(reference=w88, error in (no error)=w86) -> ()  [unwired: 1 out]
  n148 = Close Reference(reference=w89, error in (no error)=w91) -> ()  [unwired: 1 out]
  n149 = Close Reference(reference=w96, error in (no error)=w94) -> ()  [unwired: 1 out]
  n150 = Close Reference(reference=w53, error in (no error)=w51) -> ()  [unwired: 1 out]
  n151 = Close Reference(reference=w59, error in (no error)=w58) -> ()  [unwired: 1 out]
  n152 = Close Reference(reference=w61, error in (no error)=w63) -> ()  [unwired: 1 out]
  n153 = Close Reference(reference=w68, error in (no error)=w66) -> ()  [unwired: 1 out]
  n154 = Close Reference(reference=w69, error in (no error)=w71) -> ()  [unwired: 1 out]
  n155 = Close Reference(reference=w75, error in (no error)=w74) -> ()  [unwired: 1 out]
  n156 = Close Reference(reference=w79, error in (no error)=w80) -> ()  [unwired: 1 out]
  n157 = Close Reference(reference=w78, error in (no error)=w77) -> ()  [unwired: 1 out]
  n158 = Close Reference(reference=w44, error in (no error)=w45) -> ()  [unwired: 1 out]
  n159 = Close Reference(reference=w229, error in (no error)=w235) -> ()  [unwired: 1 out]
  n160 = Close Reference(reference=w60, error in (no error)=w55) -> ()  [unwired: 1 out]
  n161 = Close Reference(reference=w7, error in (no error)=w8) -> ()  [unwired: 1 out]
  n162 = Close Reference(reference=w265, error in (no error)=w267) -> ()  [unwired: 1 out]
  n163 = Close Reference(reference=w250, error in (no error)=w253) -> ()  [unwired: 1 out]
  n164 = Close Reference(reference=w249, error in (no error)=w256) -> ()  [unwired: 1 out]
  n165 = Close Reference(reference=w313, error in (no error)=w314) -> ()  [unwired: 1 out]
  n166 = Close Reference(reference=w204, error in (no error)=w286) -> ()  [unwired: 1 out]
  n167 = Close Reference(reference=w264, error in (no error)=w262) -> ()  [unwired: 1 out]
  n168 = Close Reference(reference=w251, error in (no error)=w259) -> ()  [unwired: 1 out]
  n169 = Close Reference(reference=w310, error in (no error)=w309) -> ()  [unwired: 1 out]
  n170 = Close Reference(reference=w302, error in (no error)=w301) -> ()  [unwired: 1 out]
  n171 = Close Reference(reference=w292, error in (no error)=w298) -> ()  [unwired: 1 out]
  n172 = Close Reference(reference=w289, error in (no error)=w290) -> ()  [unwired: 1 out]
  n173 = Close Reference(reference=w281, error in (no error)=w283) -> ()  [unwired: 1 out]
  n174 = Close Reference(reference=w280, error in (no error)=w278) -> ()  [unwired: 1 out]
  n175 = Close Reference(reference=w273, error in (no error)=w275) -> ()  [unwired: 1 out]
  n176 = Close Reference(reference=w272, error in (no error)=w270) -> ()  [unwired: 1 out]
  n177 = Close Reference(reference=w305, error in (no error)=w306) -> ()  [unwired: 1 out]
  n178 = Close Reference(reference=w295, error in (no error)=w294) -> ()  [unwired: 1 out]
  n179 = Number To Fractional String(number=w231, precision (6)=w4) -> (F-format string=w206:string)  [unwired: 2 in]
  n180 = Number To Fractional String(number=w177, precision (6)=w4) -> (F-format string=w162:string)  [unwired: 2 in]
  n181 = Number To Fractional String(number=w172, precision (6)=w4) -> (F-format string=w161:string)  [unwired: 2 in]
  n182 = Number To Fractional String(number=w169, precision (6)=w4) -> (F-format string=w160:string)  [unwired: 2 in]
  n183 = Number To Fractional String(number=w164, precision (6)=w4) -> (F-format string=w159:string)  [unwired: 2 in]
  n184 = Number To Fractional String(number=w87, precision (6)=w4) -> (F-format string=w84:string)  [unwired: 2 in]
  n185 = Number To Fractional String(number=w90, precision (6)=w4) -> (F-format string=w83:string)  [unwired: 2 in]
  n186 = Number To Fractional String(number=w95, precision (6)=w4) -> (F-format string=w82:string)  [unwired: 2 in]
  n187 = Number To Fractional String(number=w1, precision (6)=w4) -> (F-format string=w18:string)  [unwired: 2 in]
  n188 = Number To Fractional String(number=w62, precision (6)=w4) -> (F-format string=w17:string)  [unwired: 2 in]
  n189 = Number To Fractional String(number=w67, precision (6)=w4) -> (F-format string=w16:string)  [unwired: 2 in]
  n190 = Number To Fractional String(number=w70, precision (6)=w4) -> (F-format string=w15:string)  [unwired: 2 in]
  n191 = Number To Fractional String(number=w26, precision (6)=w4) -> (F-format string=w14:string)  [unwired: 2 in]
  n192 = Number To Fractional String(number=w25, precision (6)=w4) -> (F-format string=w13:string)  [unwired: 2 in]
  n193 = Number To Fractional String(number=w24, precision (6)=w4) -> (F-format string=w12:string)  [unwired: 2 in]
  n194 = Number To Fractional String(number=w23, precision (6)=w4) -> (F-format string=w11:string)  [unwired: 2 in]
  n195 = Number To Fractional String(number=w21, precision (6)=w4) -> (F-format string=w10:string)  [unwired: 2 in]
  n196 = Number To Fractional String(number=w312, precision (6)=w4) -> (F-format string=w227:string)  [unwired: 2 in]
  n197 = Number To Fractional String(number=w311, precision (6)=w4) -> (F-format string=w226:string)  [unwired: 2 in]
  n198 = Number To Fractional String(number=w303, precision (6)=w4) -> (F-format string=w225:string)  [unwired: 2 in]
  n199 = Number To Fractional String(number=w304, precision (6)=w4) -> (F-format string=w224:string)  [unwired: 2 in]
  n200 = Number To Fractional String(number=w297, precision (6)=w4) -> (F-format string=w223:string)  [unwired: 2 in]
  n201 = Number To Fractional String(number=w296, precision (6)=w4) -> (F-format string=w222:string)  [unwired: 2 in]
  n202 = Number To Fractional String(number=w287, precision (6)=w4) -> (F-format string=w221:string)  [unwired: 2 in]
  n203 = Number To Fractional String(number=w288, precision (6)=w4) -> (F-format string=w220:string)  [unwired: 2 in]
  n204 = Number To Fractional String(number=w284, precision (6)=w4) -> (F-format string=w219:string)  [unwired: 2 in]
  n205 = Number To Fractional String(number=w277, precision (6)=w4) -> (F-format string=w218:string)  [unwired: 2 in]
  n206 = Number To Fractional String(number=w276, precision (6)=w4) -> (F-format string=w217:string)  [unwired: 2 in]
  n207 = Number To Fractional String(number=w269, precision (6)=w4) -> (F-format string=w216:string)  [unwired: 2 in]
  n208 = Number To Fractional String(number=w268, precision (6)=w4) -> (F-format string=w215:string)  [unwired: 2 in]
  n209 = Number To Fractional String(number=w261, precision (6)=w4) -> (F-format string=w214:string)  [unwired: 2 in]
  n210 = Number To Fractional String(number=w260, precision (6)=w4) -> (F-format string=w213:string)  [unwired: 2 in]
  n211 = Number To Fractional String(number=w254, precision (6)=w4) -> (F-format string=w212:string)  [unwired: 2 in]
  n212 = Number To Fractional String(number=w255, precision (6)=w4) -> (F-format string=w211:string)  [unwired: 2 in]
  n213 = Number To Fractional String(number=w244, precision (6)=w4) -> (F-format string=w210:string)  [unwired: 2 in]
  n214 = Number To Fractional String(number=w243, precision (6)=w4) -> (F-format string=w209:string)  [unwired: 2 in]
  n215 = Number To Fractional String(number=w238, precision (6)=w4) -> (F-format string=w208:string)  [unwired: 2 in]
  n216 = Number To Fractional String(number=w236, precision (6)=w4) -> (F-format string=w207:string)  [unwired: 2 in]
  n217 = Number To Fractional String(number=w52, precision (6)=w4) -> (F-format string=w20:string)  [unwired: 2 in]
  n218 = Number To Fractional String(number=w54, precision (6)=w4) -> (F-format string=w19:string)  [unwired: 2 in]
  n219 = Number To Fractional String(number=w5, precision (6)=w4) -> (F-format string=w3:string)  [unwired: 2 in]
  n220 = Insert Into Array(array=string[] [], new element #1=w227, new element #2=w226, new element #3=w225, new element #4=w224, new element #5=w223, new element #6=w222, new element #7=w221, new element #8=w220, new element #9=w219, new element #10=w218, new element #11=w217, new element #12=w216, new element #13=w215, new element #14=w214, new element #15=w213, new element #16=w212, new element #17=w211, new element #18=w210, new element #19=w209, new element #20=w208, new element #21=w207, new element #22=w206, new element #23=w162, new element #24=w161, new element #25=w160, new element #26=w159, new element #27=w84, new element #28=w83, new element #29=w82, new element #30=w20, new element #31=w19, new element #32=w18, new element #33=w17, new element #34=w16, new element #35=w15, new element #36=w14, new element #37=w13, new element #38=w12, new element #39=w11, new element #40=w10, new element #41=w3) -> (w205:string[])  [unwired: 1 in]
  n221 = for {
    tunnel: w381 -> [w403]
    tunnel: "CONFIG PARAMETER" ("WRITE /READ SECTION") -> [w402]
    tunnel: [w401] -> w379
    tunnel: string[] ["Sway PPR", "Sway Pitch", "Surge PPR", "Surge Pitch", "Heave PPR", "Heave Pitch", "Heave distance (mm)", "Surge distance (mm)", "Sway distance (mm)", "DataSavingLoopDelay(ms)", "Acoustic Emission:", "RotHomeSurgeOffsetCounts", "RotHomeSwayOffsetCounts", "TracHomeSurgeOffsetCounts 20MM", "TracHomeSwayOffsetCounts 20MM", "TracHomeSurgeOffsetCounts 10MM", "TracHomeSwayOffsetCounts 10MM", "LRMHomeSurgeOffsetCounts", "LRMHomeSwayOffsetCounts", "Filter% ", "Filter% 2", "SAMPLES", "Heave Loop Delay", "Heave PID Speed", "Surge Jog Speed", "Heave Jog Speed", "Sway Loop Delay", "Sway Pid Speed", "Sway Jog Speed", "Depth Trip Value", "Load Trip Value", "Depth Trip Enable", "Cyclic FF Trip Value", "FF Trip Value", "Cyclic Cof Trip Value", "Cyclic FF Trip Enable", "FF Trip Enable", "Cof Trip Enable", "Load Trip Enable", "Cyclic Cof Trip Enable"] -> [w399] mode=indexing
    tunnel: w205 -> [w397] mode=indexing
    n222 = call "CONFIG FILE MAIN Unitest.vi"("WRITE /READ SECTION"=w402, "WRITE KEY"=w399, "WRITE VALUE"=w397, "error in"=w403, "PARAMETER/CONFIG"=TRUE, "Config Enum"=Config_file__FGV_Unitest_enum."WRITE") -> ("error out"=w401:errorcluster)  [unwired: 12 in, 1 out]
  }
  n223 = Unbundle By Name("main ref") -> ("About Screen.Humidity Port:"=w202:refnum<vi>)
  n224 = Unbundle By Name("main ref") -> ("About Screen.Temp Modbus:"=w197:refnum<vi>)
  n225 = Unbundle By Name("main ref") -> ("About Screen.Heave and Surge COM Port:"=w194:refnum<vi>)
  n226 = Unbundle By Name("main ref") -> ("About Screen.Sway COM Port:"=w190:refnum<vi>)
  n227 = Unbundle By Name("main ref") -> ("About Screen.Ramp Port:"=w189:refnum<vi>)
  n228 = Unbundle By Name("main ref") -> ("About Screen.ECR Port:"=w186:refnum<vi>)
  n229 = Unbundle By Name("main ref") -> ("New PID LOGIC.PID SDelay"=w152:refnum<vi>)
  n230 = Unbundle By Name("main ref") -> ("New PID LOGIC.Kp"=w151:refnum<vi>)
  n231 = Unbundle By Name("main ref") -> ("New PID LOGIC.Ki"=w146:refnum<vi>)
  n232 = Unbundle By Name("main ref") -> ("New PID LOGIC.Kd"=w145:refnum<vi>)
  n233 = Unbundle By Name("main ref") -> ("New PID LOGIC.Deadband"=w141:refnum<vi>)
  n234 = Unbundle By Name("main ref") -> ("New PID LOGIC.pct_scale"=w140:refnum<vi>)
  n235 = Unbundle By Name("main ref") -> ("New PID LOGIC.Init Step"=w137:refnum<vi>)
  n236 = Unbundle By Name("main ref") -> ("New PID LOGIC.i_limit"=w136:refnum<vi>)
  n237 = Unbundle By Name("main ref") -> ("New PID LOGIC.Max Step Linit"=w133:refnum<vi>)
  n238 = Unbundle By Name("main ref") -> ("New PID LOGIC.Max_pos_limit"=w131:refnum<vi>)
  n239 = Unbundle By Name("main ref") -> ("New PID LOGIC.Min_pos_limit"=w130:refnum<vi>)
  n240 = property class="VISAName"(reference=w202) -> (reference out=w200:refnum<vi>, error out=w201:errorcluster, "Value"=w196:refnum<visa-resource-name>)  [unwired: 1 in]
  n241 = property class="VISAName"(reference=w197) -> (reference out=w199:refnum<vi>, error out=w198:errorcluster, "Value"=w195:refnum<visa-resource-name>)  [unwired: 1 in]
  n242 = property class="VISAName"(reference=w194) -> (reference out=w192:refnum<vi>, error out=w193:errorcluster, "Value"=w185:refnum<visa-resource-name>)  [unwired: 1 in]
  n243 = property class="VISAName"(reference=w190) -> (reference out=w184:refnum<vi>, error out=w191:errorcluster, "Value"=w183:refnum<visa-resource-name>)  [unwired: 1 in]
  n244 = property class="VISAName"(reference=w189) -> (reference out=w180:refnum<vi>, error out=w188:errorcluster, "Value"=w182:refnum<visa-resource-name>)  [unwired: 1 in]
  n245 = property class="VISAName"(reference=w186) -> (reference out=w179:refnum<vi>, error out=w187:errorcluster, "Value"=w181:refnum<visa-resource-name>)  [unwired: 1 in]
  n246 = Close Reference(reference=w200, error in (no error)=w201) -> ()  [unwired: 1 out]
  n247 = Close Reference(reference=w199, error in (no error)=w198) -> ()  [unwired: 1 out]
  n248 = Close Reference(reference=w192, error in (no error)=w193) -> ()  [unwired: 1 out]
  n249 = Close Reference(reference=w184, error in (no error)=w191) -> ()  [unwired: 1 out]
  n250 = Close Reference(reference=w180, error in (no error)=w188) -> ()  [unwired: 1 out]
  n251 = Close Reference(reference=w179, error in (no error)=w187) -> ()  [unwired: 1 out]
  n252 = property class="DigNum (strict)"(reference=w152) -> (reference out=w154:refnum<vi>, error out=w153:errorcluster, "Value"=w121:dbl)  [unwired: 1 in]
  n253 = property class="DigNum (strict)"(reference=w151) -> (reference out=w149:refnum<vi>, error out=w150:errorcluster, "Value"=w120:dbl)  [unwired: 1 in]
  n254 = property class="DigNum (strict)"(reference=w146) -> (reference out=w148:refnum<vi>, error out=w147:errorcluster, "Value"=w119:dbl)  [unwired: 1 in]
  n255 = property class="DigNum (strict)"(reference=w145) -> (reference out=w143:refnum<vi>, error out=w144:errorcluster, "Value"=w118:dbl)  [unwired: 1 in]
  n256 = property class="DigNum (strict)"(reference=w141) -> (reference out=w127:refnum<vi>, error out=w142:errorcluster, "Value"=w117:dbl)  [unwired: 1 in]
  n257 = property class="DigNum (strict)"(reference=w140) -> (reference out=w128:refnum<vi>, error out=w139:errorcluster, "Value"=w116:dbl)  [unwired: 1 in]
  n258 = property class="DigNum (strict)"(reference=w137) -> (reference out=w126:refnum<vi>, error out=w138:errorcluster, "Value"=w115:dbl)  [unwired: 1 in]
  n259 = property class="DigNum (strict)"(reference=w136) -> (reference out=w125:refnum<vi>, error out=w135:errorcluster, "Value"=w114:dbl)  [unwired: 1 in]
  n260 = property class="DigNum (strict)"(reference=w133) -> (reference out=w124:refnum<vi>, error out=w134:errorcluster, "Value"=w113:dbl)  [unwired: 1 in]
  n261 = property class="DigNum (strict)"(reference=w131) -> (reference out=w123:refnum<vi>, error out=w132:errorcluster, "Value"=w112:dbl)  [unwired: 1 in]
  n262 = property class="DigNum (strict)"(reference=w130) -> (reference out=w122:refnum<vi>, error out=w129:errorcluster, "Value"=w111:dbl)  [unwired: 1 in]
  n263 = Insert Into Array(array=string[] [], new element #1=w196, new element #2=w195, new element #3=w185, new element #4=w183, new element #5=w182, new element #6=w181) -> (w375:string[])  [unwired: 1 in]
  n264 = for {
    tunnel: w379 -> [w410]
    tunnel: "COM PORT" ("WRITE /READ SECTION") -> [w409]
    tunnel: [w408] -> w156
    tunnel: string[] ["HUMIDITY PORT", "TEMP MODBUS", "HEAVE AND SURGE COM PORT", "SWAY COM PORT", "RAMP PORT", "ECR PORT"] -> [w406] mode=indexing
    tunnel: w375 -> [w405] mode=indexing
    n265 = call "CONFIG FILE MAIN Unitest.vi"("WRITE /READ SECTION"=w409, "WRITE KEY"=w406, "WRITE VALUE"=w405, "error in"=w410, "PARAMETER/CONFIG"=TRUE, "Config Enum"=Config_file__FGV_Unitest_enum."WRITE") -> ("error out"=w408:errorcluster)  [unwired: 12 in, 1 out]
  }
  n266 = Close Reference(reference=w154, error in (no error)=w153) -> ()  [unwired: 1 out]
  n267 = Close Reference(reference=w149, error in (no error)=w150) -> ()  [unwired: 1 out]
  n268 = Close Reference(reference=w148, error in (no error)=w147) -> ()  [unwired: 1 out]
  n269 = Close Reference(reference=w143, error in (no error)=w144) -> ()  [unwired: 1 out]
  n270 = Close Reference(reference=w127, error in (no error)=w142) -> ()  [unwired: 1 out]
  n271 = Close Reference(reference=w128, error in (no error)=w139) -> ()  [unwired: 1 out]
  n272 = Close Reference(reference=w126, error in (no error)=w138) -> ()  [unwired: 1 out]
  n273 = Close Reference(reference=w125, error in (no error)=w135) -> ()  [unwired: 1 out]
  n274 = Close Reference(reference=w124, error in (no error)=w134) -> ()  [unwired: 1 out]
  n275 = Close Reference(reference=w123, error in (no error)=w132) -> ()  [unwired: 1 out]
  n276 = Close Reference(reference=w122, error in (no error)=w129) -> ()  [unwired: 1 out]
  n277 = Number To Fractional String(number=w121, precision (6)=w110) -> (F-format string=w108:string)  [unwired: 2 in]
  n278 = Number To Fractional String(number=w120, precision (6)=w110) -> (F-format string=w107:string)  [unwired: 2 in]
  n279 = Number To Fractional String(number=w119, precision (6)=w110) -> (F-format string=w106:string)  [unwired: 2 in]
  n280 = Number To Fractional String(number=w118, precision (6)=w110) -> (F-format string=w105:string)  [unwired: 2 in]
  n281 = Number To Fractional String(number=w117, precision (6)=w110) -> (F-format string=w104:string)  [unwired: 2 in]
  n282 = Number To Fractional String(number=w116, precision (6)=w110) -> (F-format string=w103:string)  [unwired: 2 in]
  n283 = Number To Fractional String(number=w115, precision (6)=w110) -> (F-format string=w102:string)  [unwired: 2 in]
  n284 = Number To Fractional String(number=w114, precision (6)=w110) -> (F-format string=w101:string)  [unwired: 2 in]
  n285 = Number To Fractional String(number=w113, precision (6)=w110) -> (F-format string=w100:string)  [unwired: 2 in]
  n286 = Number To Fractional String(number=w112, precision (6)=w110) -> (F-format string=w99:string)  [unwired: 2 in]
  n287 = Number To Fractional String(number=w111, precision (6)=w110) -> (F-format string=w98:string)  [unwired: 2 in]
  n288 = Insert Into Array(array=string[] [], new element #1=w108, new element #2=w107, new element #3=w106, new element #4=w105, new element #5=w104, new element #6=w103, new element #7=w102, new element #8=w101, new element #9=w100, new element #10=w99, new element #11=w98) -> (w97:string[])  [unwired: 1 in]
  n289 = for {
    tunnel: w156 -> [w417]
    tunnel: "NEW PID PARAMETERS" ("WRITE /READ SECTION") -> [w416]
    tunnel: [w415] -> w157
    tunnel: string[] ["PID DELAY (sec)", "Kp", "Ki", "Kd", "Deaadband", "pct_scale", "Init_step", "i_limit", "Max Step Limit", "Min_pos_limit", "Max_pos_limit", "Fine_tune_zone"] -> [w413] mode=indexing
    tunnel: w97 -> [w411] mode=indexing
    n290 = call "CONFIG FILE MAIN Unitest.vi"("WRITE /READ SECTION"=w416, "WRITE KEY"=w413, "WRITE VALUE"=w411, "error in"=w417, "PARAMETER/CONFIG"=TRUE, "Config Enum"=Config_file__FGV_Unitest_enum."WRITE") -> ("error out"=w415:errorcluster)  [unwired: 12 in, 1 out]
  }
  n291 = call "CONFIG FILE MAIN Unitest.vi"("error in"=w157, "Config Enum"=Config_file__FGV_Unitest_enum."CLOSE") -> ("error out"=→"error out":errorcluster)  [unwired: 16 in, 1 out]
